vi "Test String Functions.vi"() -> ()   [LabVIEW 2021]
uses:
  Source/Abs_Types/String/Simple Read.vi
  Source/Abs_Types/I32 Integer/Simple Read.vi
  Source/Abs_Types/I32 Integer/Abs_I32 Integer.lvclass
  C:/Program Files (x86)/National Instruments/LabVIEW 2021/vi.lib/TSA/Abstract Data Classes/Abs_Types/Numeric/Abs_Numeric.lvclass
  C:/Program Files (x86)/National Instruments/LabVIEW 2021/vi.lib/TSA/Abstract Data Classes/Abs_Types/Value/Abs_Value.lvclass
  Source/Abs_Types/String/Abs_String.lvclass
  Source/Functions/Conversion/Support/DBL/ConvertTo_DBL.lvclass
  Source/Constants/Support/Str/Str.vi
  Source/Functions/Conversion/Support/DBL/Method.vi
  Source/Functions/Math/Support/Decrement/I32/Method.vi
  Source/Constants/Support/I32/I32.vi
  Source/Constants/Support/Str/Const_Str.lvclass
  Source/Functions/Math/Support/Decrement/I32/Decrement_I32.lvclass
  Source/Constants/Support/I32/Const_I32.lvclass
  C:/TSA/LV_Abstract/Source/Abs_Types/Integer/Abs_Integer.lvclass
  C:/Program Files (x86)/National Instruments/LabVIEW 2021/vi.lib/TSA/Abstract Data Classes/Abs_Types/Type/Abs_Type.lvclass
  C:/TSA/LV_Abstract/Source/Abs_Types/I32 Integer/Abs_I32 Integer.lvclass
panel:
  out "String 4":string
  out "String 3":string
  out "String 2":string
  out "String":string
  out "Lenght":i32
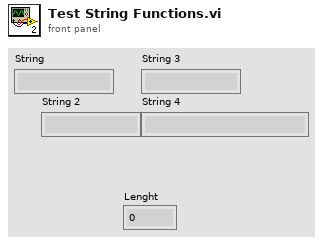
[diagram p1: front panel]
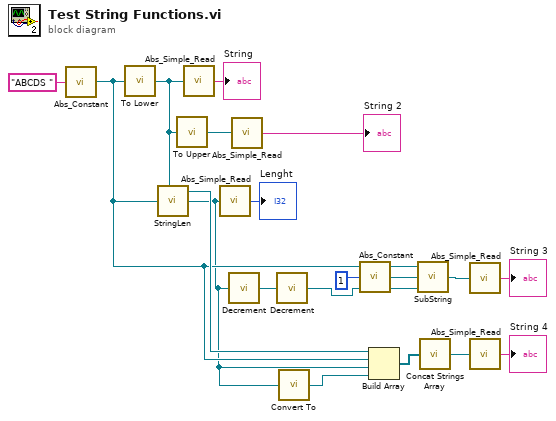
[diagram p0: block diagram]
diagram:
  n1 = call-poly "Abs_Constant.vi"("String"="ABCDS ") -> ("Abs_String.lvclass"=w5:refnum<class "Abs_String.lvclass">)  [unwired: 4 in]
  n2 = call "To Lower.vi"("String"=w5) -> ("Result"=w6:refnum<class "Abs_String.lvclass">)  [unwired: 4 in]
  n3 = call "StringLen.vi"("String"=w5) -> ("Result"=w2:refnum<class "Abs_I32 Integer.lvclass">)  [unwired: 4 in]
  n4 = call "To Upper.vi"("String"=w6) -> ("Result"=w14:refnum<class "Abs_String.lvclass">)  [unwired: 4 in]
  n5 = call-poly "Abs_Simple_Read.vi"("Abs_String in"=w6) -> ("String"=→"String":string)  [unwired: 4 in]
  n6 = call-poly "Abs_Simple_Read.vi"("Class"=w2) -> ("Value"=→"Lenght":i32)  [unwired: 4 in]
  n7 = call-poly "Decrement.vi"("Value"=w2) -> ("Result"=w9:refnum<class "Abs_I32 Integer.lvclass">)  [unwired: 4 in]
  n8 = call-poly "Abs_Simple_Read.vi"("Abs_String in"=w14) -> ("String"=→"String 2":string)  [unwired: 4 in]
  n9 = call-poly "Decrement.vi"("Value"=w9) -> ("Result"=w8:refnum<class "Abs_I32 Integer.lvclass">)  [unwired: 4 in]
  n10 = call-poly "Convert To.vi"("Value"=w2) -> ("Result"=w1:refnum<class "ConvertTo_DBL.lvclass">)  [unwired: 4 in]
  n11 = call-poly "Abs_Constant.vi"("Value"=1) -> ("Constant"=w10:refnum<class "Abs_I32 Integer.lvclass">)  [unwired: 4 in]
  n12 = Build Array(w6, w5, w2, w1) -> (w7:refnum<class "Abs_Value.lvclass">[])
  n13 = call "SubString.vi"("Length"=w8, "Offset"=w10, "String"=w5) -> ("Result"=w12:refnum<class "Abs_String.lvclass">)
  n14 = call "Concat Strings Array.vi"("Strings"=w7) -> ("Result"=w4:refnum<class "Abs_String.lvclass">)  [unwired: 4 in]
  n15 = call-poly "Abs_Simple_Read.vi"("Abs_String in"=w12) -> ("String"=→"String 3":string)  [unwired: 4 in]
  n16 = call-poly "Abs_Simple_Read.vi"("Abs_String in"=w4) -> ("String"=→"String 4":string)  [unwired: 4 in]
